vi "Run Script w_Script Triggers.vi"(5 "Total_Num_Script_Triggers":i32=1, 7 "script name":string="Cmax", 8 "error in (no error)":errorcluster, 10 "Delay Between triggers":dbl=0.001 caption="Delay Time (s)" format="%#_6p", 11 "Semiconductor Module Context":T1) -> (0 "error out":errorcluster)   [LabVIEW 2013]
uses:
  <vilib>/NI_TestStand_SemiconductorModule/NI_TestStand_Semiconductor_Module.lvlibp/PinMap/General/SemiconductorModuleContext.ctl
  <instrlib>/niHSDIO/niHSDIO.llb/niHSDIO_ctl Trigger Script - trigID Values (Ring).ctl
  <vilib>/NI_TestStand_SemiconductorModule/NI_TestStand_Semiconductor_Module.lvlibp
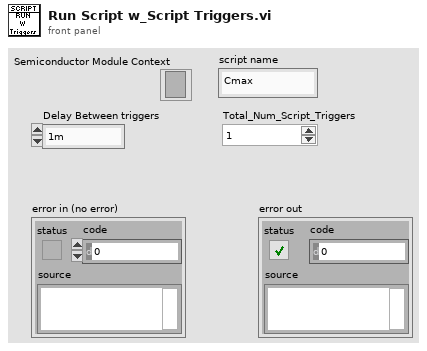
[diagram p1: front panel]
types:
  T1 = typedef "NI_TestStand_Semiconductor_Module.lvlibp/SemiconductorModuleContext.ctl" = refnum<k7>
  T2 = typedef "niHSDIO_ctl Trigger Script - trigID Values (Ring).ctl" = string
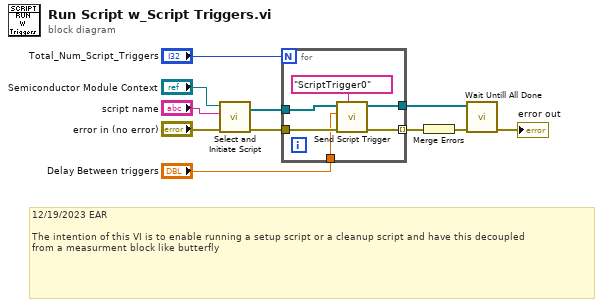
[diagram p0: block diagram]
diagram:
  # "12/19/2023 EAR\n\nThe intention of this VI is to enable running a setup script or a cleanup script and have this decoupled \nfrom a measurment block like butterfly"
  n1 = call "Select and Initiate Script.vi"("error in (no error)"="error in (no error)", "script name"="script name", "Semiconductor Module Context"="Semiconductor Module Context") -> ("error out"=w11:errorcluster, "HSDIO GEN Sessions Out"=w10:refnum<k15>[])  [unwired: 6 in, 1 out]
  n2 = for {
    N: "Total_Num_Script_Triggers" -> [_]
    tunnel: w11 -> [w16]
    tunnel: w10 -> [w15]
    tunnel: [w14] -> w8 mode=indexing
    tunnel: [w13] -> w9
    tunnel: "Delay Between triggers" -> [w12]
    n3 = call "Send Script Trigger.vi"("trigger id (script trigger 0)"=T2 "ScriptTrigger0", "error in (no error)"=w16, "Delay Time (s)"=w12, "HSDIO Sessions In"=w15) -> ("error out"=w14:errorcluster, "HSDIO Sessions Out"=w13:refnum<k15>[])  [unwired: 6 in]
  }
  n4 = Merge Errors(w8) -> (w7:errorcluster)
  n5 = call "Wait Untill All Done.vi"("error in (no error)"=w7, "HSDIO Sessions In"=w9) -> ("error out"=→"error out":errorcluster)  [unwired: 8 in, 1 out]
